vi "Set Tuner Gain.vi"(8 "error in (no error)":errorcluster, 10 "Tuner Gain":dbl, 11 "RTL-SDR in":refnum<class "Session.lvclass">) -> (0 "error out":errorcluster, 3 "RTL-SDR out":refnum<class "Session.lvclass">)   [LabVIEW 2021, in "RTL-SDR.lvlib" / "Session.lvclass"]
uses:
  Session.lvclass
  Session.lvclass/Session.ctl
  Gain Mode.ctl
  RTL-SDR.lvlib
  lib/librtlsdr.dll
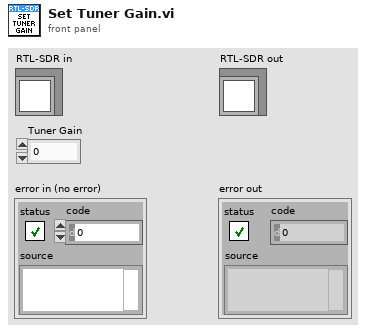
[diagram p1: front panel]
types:
  T1 = typedef "RTL-SDR.lvlib/Gain Mode.ctl" = i32
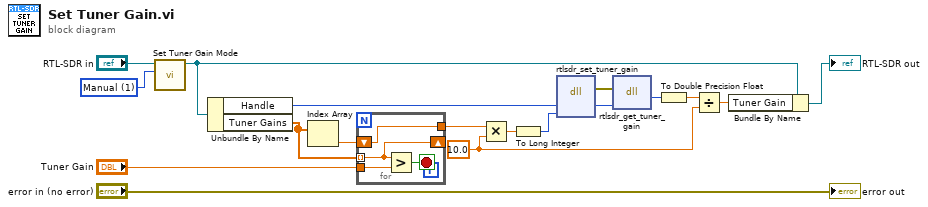
[diagram p0: block diagram]
diagram:
  w5 = T1 1 items=["Automatic", "Manual"] ("Tuner Gain Mode")
  w10 = 10.0 ("y")
  n1 = call "Set Tuner Gain Mode.vi"("Tuner Gain Mode"=w5, "RTL-SDR in"="RTL-SDR in") -> ("RTL-SDR out"=w6:refnum<class "Session.lvclass">)  [unwired: 8 in, 1 out]
  n2 = Unbundle By Name(w6) -> ("Handle"=w16:u64, "Tuner Gains"=w2:dbl[])
  n3 = Index Array(array=w2) -> (element=w1:dbl)  [unwired: 1 in]
  n4 = for {
    tunnel: "Tuner Gain" -> [w22]
    tunnel: w2 -> [w20] mode=indexing
    shift-right: [w20] -> _
    shift-left: w1 -> [w19]
    tunnel: [w19] -> w3
    stop <- w21 stop-if-true
    n5 = Greater?(x=w20, y=w22) -> (0:w21:bool)
  }
  n6 = Multiply(x=w3, y=w10) -> (x*y=w17:dbl)
  n7 = To Long Integer(number=w17) -> (32bit integer=w15:i32)
  n8 = dll-call lib="C:/dev/IlluminatedG/lv-rtl-sdr/lib/librtlsdr.dll" fn="rtlsdr_set_tuner_gain"("dev"=w16, "gain"=w15) -> (error out=w13:errorcluster, "dev"=w14:u64)  [unwired: 5 in, 1 out]
  n9 = dll-call lib="C:/dev/IlluminatedG/lv-rtl-sdr/lib/librtlsdr.dll" fn="rtlsdr_get_tuner_gain"(error in=w13, "dev"=w14) -> ("return type"=w12:i32)  [unwired: 3 in, 2 out]
  n10 = To Double Precision Float(number=w12) -> (double precision float=w11:dbl)
  n11 = Divide(x=w11, y=w10) -> (x/y=w8:dbl)
  n12 = Bundle By Name(cluster=w6, "Tuner Gain"=w8) -> (→"RTL-SDR out":refnum<class "Session.lvclass">)
  "error out" <- "error in (no error)"
